vi "Main.vi"() -> ()   [LabVIEW 2013]
doc: "This template is for the Queued Message Handler design pattern.\n\nThe Event Handling Loop generates messages based on user interface actions.\n\nThe Message Handling Loop processes messages generated by the Event Handling Loop, or by other messages. The messages are string values, so new messages can be added easily to the Message Cases case structure in the Message Handling Loop. Each message cluster can also provide an optional value for Message Data, which is a variant that can be converted to whatever message-specific data is required."
uses:
  controls/UI Data.ctl
  <vilib>/addons/zeromq/socket_type.ctl
  <vilib>/addons/zeromq/socket_options.ctl
  controls/JSON RPC Request.ctl
  controls/JSON RPC Response.ctl
  support/Message Queue/Enqueue Message (Array).vi
  support/Message Queue/Enqueue Message (Single).vi
  <vilib>/Utility/error.llb/Error Cluster From Error Code.vi
  <vilib>/ErrorRing/Error Ring.xnode
  support/Message Queue/Message Queue.lvlib
  support/User Event - Stop/User Event - Stop.lvlib
  <vilib>/addons/zeromq/zmq_context.lvclass
  <vilib>/addons/zeromq/zeromq.lvlib
  <vilib>/addons/zeromq/zmq_socket.lvclass
panel:
  out "Display <Replace Me>":string
  in  "Do Something Else <Replace Me>":bool
  in  "Do Something <Replace Me>":bool
  in  "Exit":bool
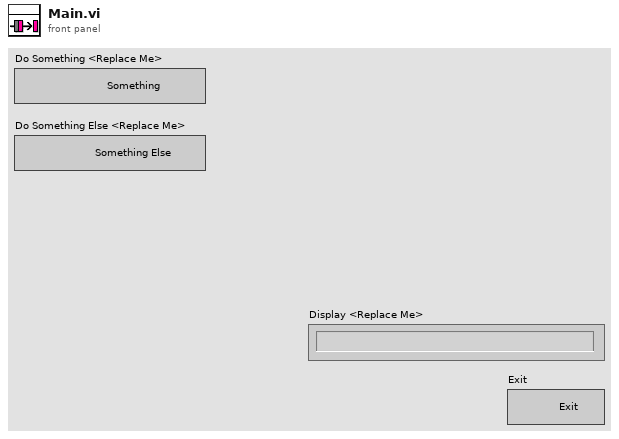
[diagram p1: front panel]
types:
  T1 = typedef "zeromq.lvlib/socket_options.ctl" = enum8{"NONE", "ZMQ_HWM", "<2>", "ZMQ_SWAP", "ZMQ_AFFINITY", "ZMQ_IDENTITY", "ZMQ_SUBSCRIBE", "ZMQ_UNSUBSCRIBE", "ZMQ_RATE", "ZMQ_RECOVERY_IVL", "ZMQ_MCAST_LOOP", "ZMQ_SNDBUF", "ZMQ_RCVBUF", "ZMQ_RCVMORE", "ZMQ_FD", "ZMQ_EVENTS", "ZMQ_TYPE", "ZMQ_LINGER", "ZMQ_RECONNECT_IVL", "ZMQ_BACKLOG", "ZMQ_RECOVERY_IVL_MSEC", "ZMQ_RECONNECT_IVL_MAX", "ZMQ_MAXMSGSIZE", "ZMQ_SNDHWM", "ZMQ_RCVHWM", "ZMQ_MULTICAST_HOPS", "<26>", "ZMQ_RCVTIMEO", "ZMQ_SNDTIMEO", "<29>", "<30>", "ZMQ_IPV4ONLY", "ZMQ_LAST_ENDPOINT", "ZMQ_ROUTER_MANDATORY", "ZMQ_TCP_KEEPALIVE", "ZMQ_TCP_KEEPALIVE_CNT", "ZMQ_TCP_KEEPALIVE_IDLE", "ZMQ_TCP_KEEPALIVE_INTVL", "ZMQ_TCP_ACCEPT_FILTER", "ZMQ_DELAY_ATTACH_ON_CONNECT", "ZMQ_XPUB_VERBOSE"}
  T2 = typedef "zeromq.lvlib/socket_type.ctl" = enum8{"ZMQ_PAIR", "ZMQ_PUB", "ZMQ_SUB", "ZMQ_REQ", "ZMQ_REP", "ZMQ_DEALER", "ZMQ_ROUTER", "ZMQ_PULL", "ZMQ_PUSH", "ZMQ_XPUB", "ZMQ_XSUB"}
  T3 = typedef "UI Data.ctl" = cluster{"Boolean <Replace Me>":bool, "String <Replace Me>":string, "Numeric <Replace Me>":dbl, "Do Something Ref":refnum<vi>, "Do Something Else Ref":refnum<vi>, "Data Display Ref":refnum<vi>, "Exit Button Ref":refnum<vi>}
  T4 = typedef "Message Queue.lvlib/All Message Queues.ctl" = cluster{"UI":refnum<queue>}
  T5 = typedef "JSON RPC Request.ctl" = cluster{"id":dbl, "method":string, "jsonrpc":string, "params":string}
  T6 = typedef "JSON RPC Response.ctl" = cluster{"id":dbl, "result":string, "jsonrpc":string}
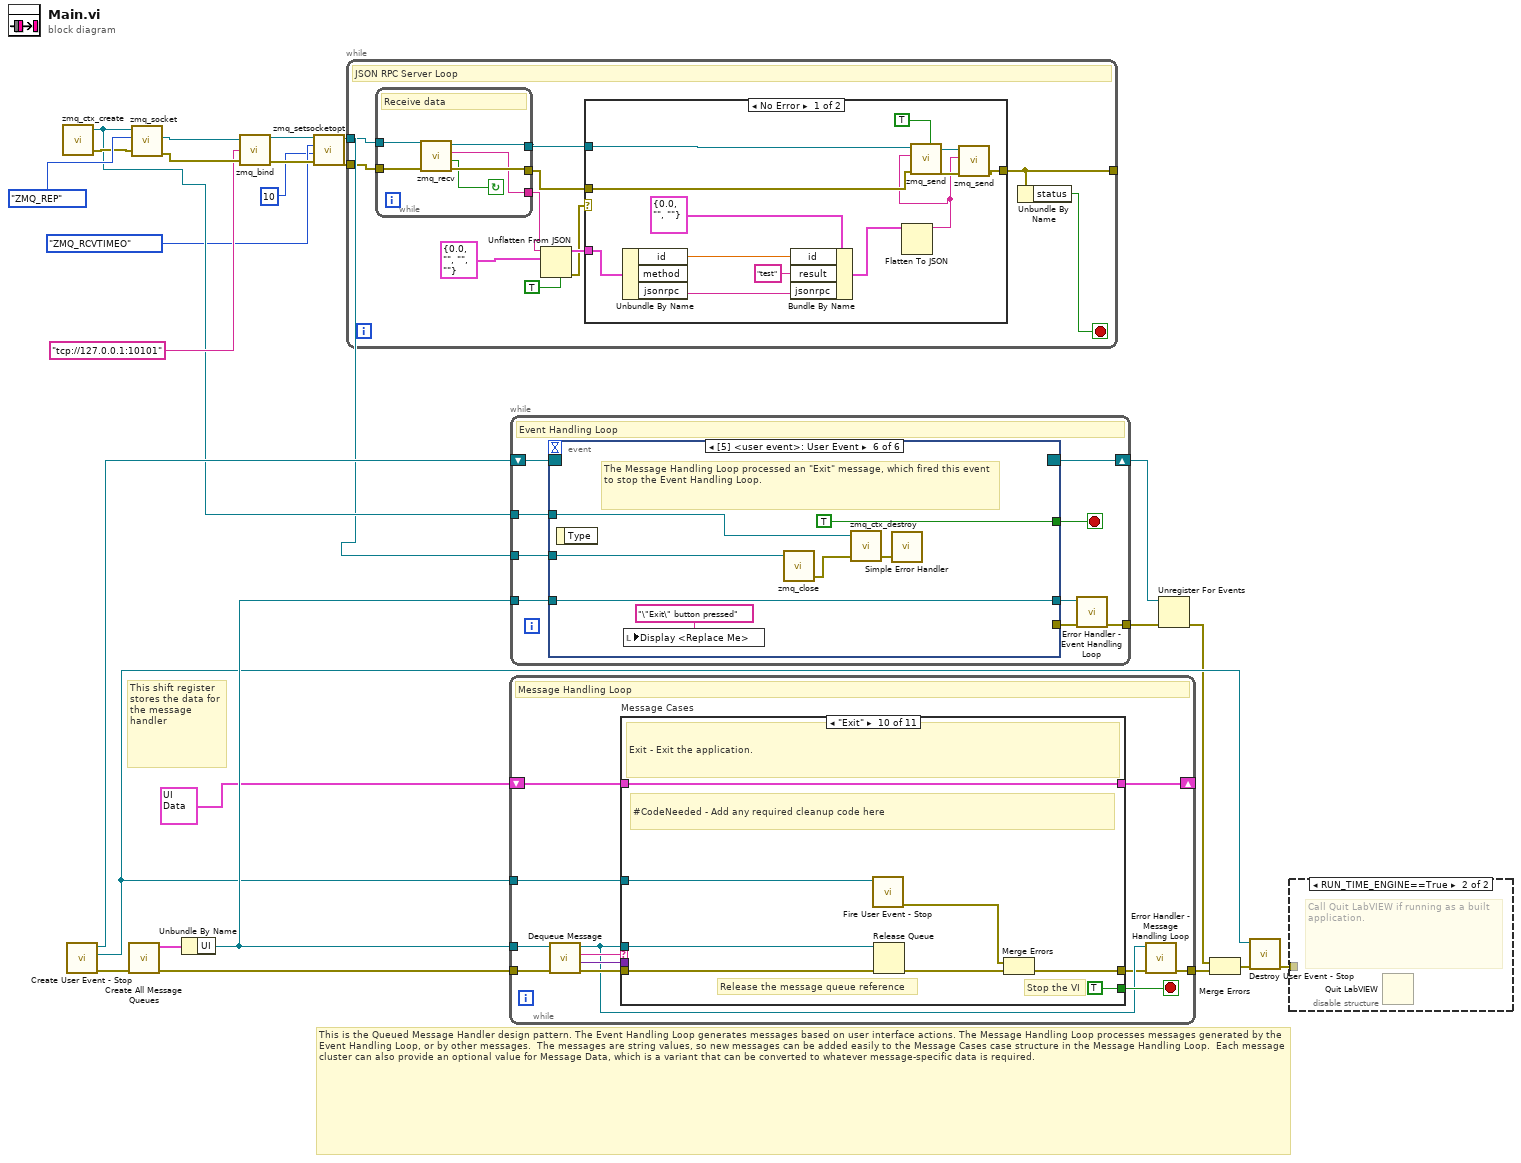
[diagram p0: block diagram]
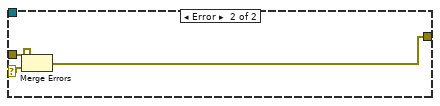
[diagram p2: hidden frame]
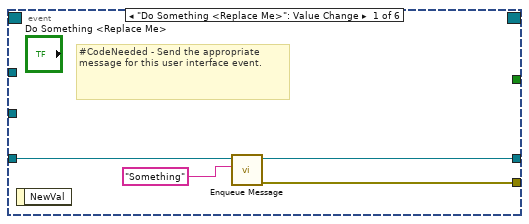
[diagram p4: hidden frame]
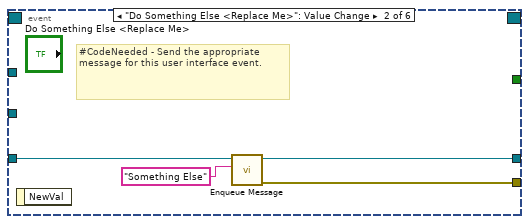
[diagram p5: hidden frame]
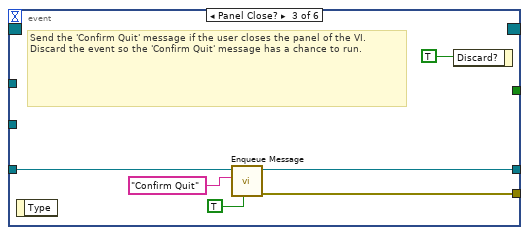
[diagram p6: hidden frame]
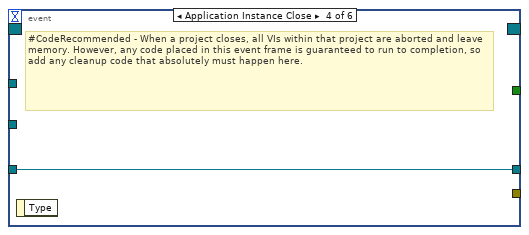
[diagram p7: hidden frame]
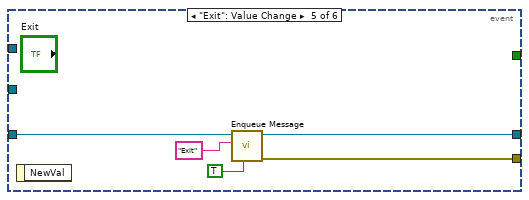
[diagram p8: hidden frame]
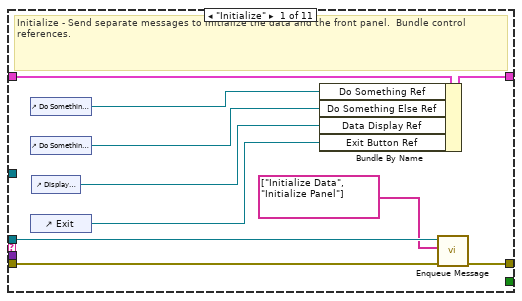
[diagram p9: hidden frame]
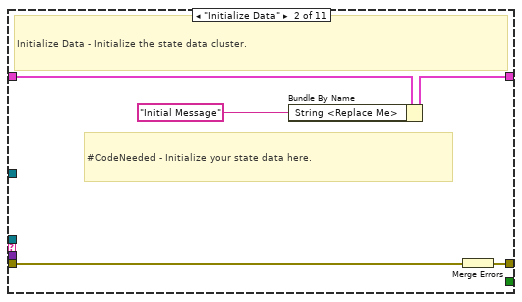
[diagram p10: hidden frame]
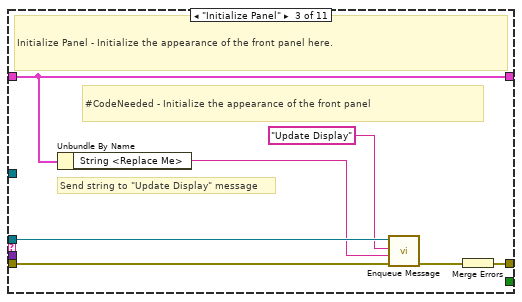
[diagram p11: hidden frame]
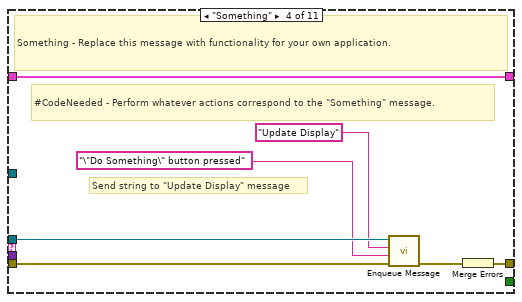
[diagram p12: hidden frame]
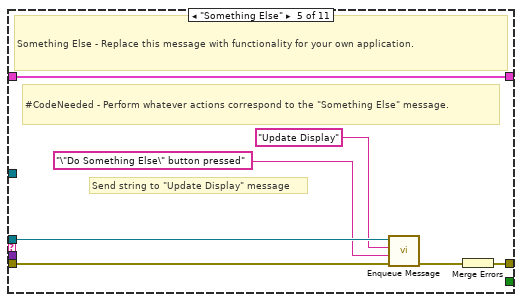
[diagram p13: hidden frame]
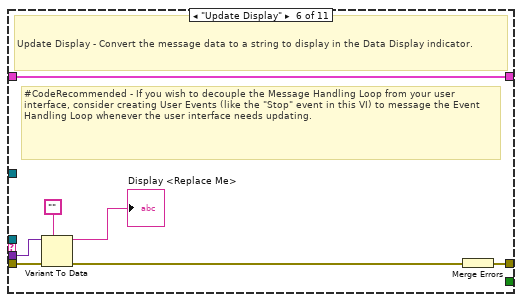
[diagram p14: hidden frame]
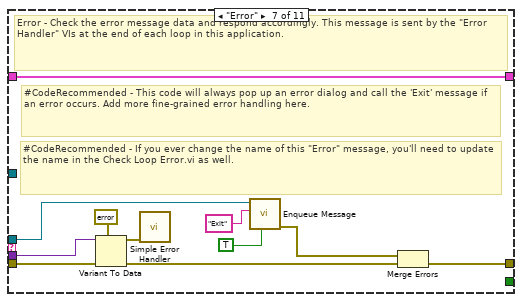
[diagram p15: hidden frame]
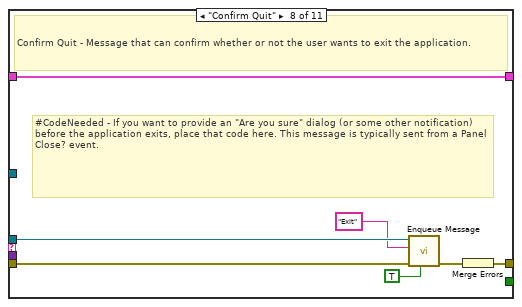
[diagram p16: hidden frame]
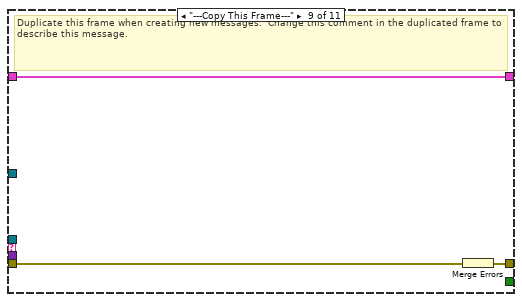
[diagram p17: hidden frame]
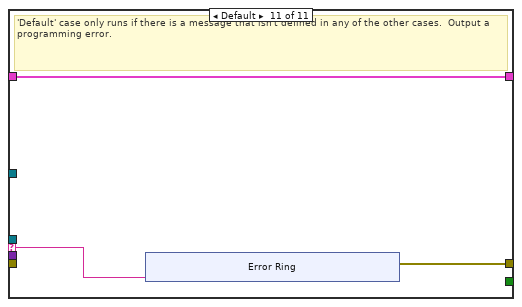
[diagram p18: hidden frame]
diagram:
  # "This is the Queued Message Handler design pattern. The Event Handling Loop generates messages based on user interface actions. The Message Handling Loop processes messages generated by the Event Handling Loop, or by other messages.  The messages are string values, so new messages can be added easily to the Message Cases case structure in the Message Handling Loop.  Each message cluster can also provide an optional value for Message Data, which is a variant that can be converted to whatever message-specific data is required."
  # "This shift register stores the data for the message handler"
  n1 = call <vilib>:"zmq_ctx_create.vi"() -> ("error out"=w11:errorcluster, "context out"=w7:refnum<class "zmq_context.lvclass">)  [unwired: 4 in]
  n2 = call "Create User Event - Stop.vi"() -> ("error out"=w20:errorcluster, "User Event - Stop"=w18:refnum<user-event>, "Stop Event Registration Refnum"=w21:refnum<event-registration>)  [unwired: 9 in]
  n3 = call "Create All Message Queues.vi"("error in (no error)"=w20) -> ("error out"=w25:errorcluster, "Message Queues out"=w24:T4)  [unwired: 9 in]
  n4 = call <vilib>:"zmq_socket.vi"("error in"=w11, "socket type"=socket_type."ZMQ_REP", "context in"=w7) -> ("error out"=w10:errorcluster, "socket out"=w9:refnum<class "zmq_socket.lvclass">)  [unwired: 2 in, 1 out]
  n5 = Unbundle By Name(w24) -> ("UI"=w22:refnum<queue>)
  n6 = call <vilib>:"zmq_bind.vi"("error in"=w10, "endpoint"="tcp://127.0.0.1:10101", "socket in"=w9) -> ("error out"=w5:errorcluster, "socket out"=w6:refnum<class "zmq_socket.lvclass">)  [unwired: 1 in]
  n7 = call <vilib>:"zmq_setsocketopt.vi"("error in"=w5, "value"=10, "option"=socket_options."ZMQ_RCVTIMEO", "socket in"=w6) -> ("error out"=w2:errorcluster, "socket out"=w1:refnum<class "zmq_socket.lvclass">)  [unwired: 2 in]
  n8 = while {
    tunnel: [w32] -> _
    tunnel: w1 -> [w35]
    tunnel: w2 -> [w34]
    stop <- w31 stop-if-true
    # "JSON RPC Server Loop"
    n9 = while {
      tunnel: [w58] -> w33
      tunnel: [w57] -> w36
      tunnel: w35 -> [w55]
      tunnel: w34 -> [w54]
      tunnel: [w53] -> w30
      stop <- w56 continue-if-true
      # "Receive data"
      n10 = call <vilib>:"zmq_recv.vi"("error in"=w54, "socket in"=w55) -> ("error out"=w58:errorcluster, "more?"=w56:bool, "data"=w53:string, "socket out"=w57:refnum<class "zmq_socket.lvclass">)  [unwired: 3 in, 1 out]
    }
    n11 = Unflatten From JSON(JSON string=w30, type and defaults=T5 {"id"=0.0, "method"="", "jsonrpc"="", "params"=""} ("JSON RPC Request"), strict validation? (F)=TRUE) -> (value=w28:T5, error out=w26:errorcluster)  [unwired: 4 in]
    n12 = case shown="No Error" w26 {
      selector: w26 -> [_ w52]
      tunnel: w36 -> [w49 _]
      tunnel: w33 -> [w48 w51]
      tunnel: [w47 w50] -> w32
      tunnel: w28 -> [w46 _]
      frame No Error {
        n13 = Unbundle By Name(w46) -> ("id"=w39:dbl, "jsonrpc"=w40:string)  [unwired: 1 out]
        n14 = Bundle By Name(cluster=T6 {"id"=0.0, "result"="", "jsonrpc"=""} ("JSON RPC Response"), "id"=w39, "result"="test", "jsonrpc"=w40) -> (w41:T6)
        n15 = Flatten To JSON(anything=w41) -> (JSON string=w37:string)  [unwired: 2 in, 1 out]
        n16 = call <vilib>:"zmq_send.vi"("error in"=w48, "data"=w37, "socket in"=w49, "more? (F)"=TRUE) -> ("error out"=w43:errorcluster, "socket out"=w44:refnum<class "zmq_socket.lvclass">)  [unwired: 3 in]
        n17 = call <vilib>:"zmq_send.vi"("error in"=w43, "data"=w37, "socket in"=w44) -> ("error out"=w47:errorcluster)  [unwired: 4 in, 1 out]
      }
      frame Error {
        n18 = Merge Errors(w51, w52) -> (w50:errorcluster)
      }
    }
    n19 = Unbundle By Name(w32) -> ("status"=w31:bool)
  }
  n20 = while {
    tunnel: w22 -> [w62]
    shift-right: [w69] -> _
    shift-left: T3 {"Boolean <Replace Me>"=FALSE, "String <Replace Me>"="", "Numeric <Replace Me>"=0.0, "Do Something Ref"=refnum, "Do Something Else Ref"=refnum, "Data Display Ref"=refnum, "Exit Button Ref"=refnum} ("Data Cluster") -> [w70]
    tunnel: w18 -> [w67]
    tunnel: w25 -> [w66]
    tunnel: [w60] -> w23
    stop <- w68 stop-if-true
    # "Message Handling Loop"
    n21 = call "Dequeue Message.vi"("error in (no error)"=w66, "Message Queue"=w62) -> ("error out"=w65:errorcluster, "Message Data"=w63:variant, "Message"=w64:string, "dup Message Queue"=w61:refnum<queue>)  [unwired: 6 in]
    n22 = case "Message Cases" shown="\"Exit\"" w64 {
      selector: w64 -> [_ _ _ _ _ _ _ _ _ _ w143]
      tunnel: w61 -> [w78 _ w89 w95 w102 _ w116 w127 _ w142 _]
      tunnel: w65 -> [w79 w85 w90 w97 w104 w111 w124 w131 w134 w137 _]
      tunnel: [w80 w81 w91 w98 w105 w112 w117 w129 w132 w138 w144] -> w59
      tunnel: w70 -> [w77 w84 w92 w99 w106 w113 w123 w130 w133 w141 w145]
      tunnel: [w76 w83 w92 w99 w106 w113 w123 w130 w133 w141 w145] -> w69
      tunnel: [_ _ _ _ _ _ _ _ _ TRUE _] -> w68
      tunnel: w63 -> [_ _ _ _ _ w110 w122 _ _ _ _]
      tunnel: w67 -> [_ _ _ _ _ _ _ _ _ w136 _]
      frame "Initialize" {
        # "Initialize - Send separate messages to initialize the data and the front panel.  Bundle control references."
        n23 = control-ref of="Do Something <Replace Me>"() -> (w75:refnum<vi>)
        n24 = control-ref of="Do Something Else <Replace Me>"() -> (w74:refnum<vi>)
        n25 = control-ref of="Exit"() -> (w72:refnum<vi>)
        n26 = control-ref of="Display <Replace Me>"() -> (w73:refnum<vi>)
        n27 = Bundle By Name(cluster=w77, "Do Something Ref"=w75, "Do Something Else Ref"=w74, "Data Display Ref"=w73, "Exit Button Ref"=w72) -> (w76:T3)
        n28 = call-poly "Enqueue Message.vi"("error in (no error)"=w79, "Message Array"=string[] ["Initialize Data", "Initialize Panel"], "Message Queue"=w78) -> ("error out"=w80:errorcluster)  [unwired: 7 in, 1 out]
      }
      frame "Initialize Data" {
        # "#CodeNeeded - Initialize your state data here."
        # "Initialize Data - Initialize the state data cluster."
        n29 = Bundle By Name(cluster=w84, "String <Replace Me>"="Initial Message" ("Initial Message")) -> (w83:T3)
        n30 = Merge Errors(w85) -> (w81:errorcluster)
      }
      frame "Initialize Panel" {
        # "Send string to \"Update Display\" message"
        # "#CodeNeeded - Initialize the appearance of the front panel"
        # "Initialize Panel - Initialize the appearance of the front panel here."
        n31 = Unbundle By Name(w92) -> ("String <Replace Me>"=w86:string)
        n32 = call-poly "Enqueue Message.vi"("error in (no error)"=w90, "Message Data"=w86, "Message"="Update Display", "Message Queue"=w89) -> ("error out"=w88:errorcluster)  [unwired: 6 in, 1 out]
        n33 = Merge Errors(w88) -> (w91:errorcluster)
      }
      frame "Something" {
        # "Send string to \"Update Display\" message"
        # "#CodeNeeded - Perform whatever actions correspond to the \"Something\" message."
        # "Something - Replace this message with functionality for your own application."
        n34 = call-poly "Enqueue Message.vi"("error in (no error)"=w97, "Message Data"="\"Do Something\" button pressed" ("\"Do Something\" button pressed"), "Message"="Update Display", "Message Queue"=w95) -> ("error out"=w96:errorcluster)  [unwired: 6 in, 1 out]
        n35 = Merge Errors(w96) -> (w98:errorcluster)
      }
      frame "Something Else" {
        # "Send string to \"Update Display\" message"
        # "#CodeNeeded - Perform whatever actions correspond to the \"Something Else\" message."
        # "Something Else - Replace this message with functionality for your own application."
        n36 = call-poly "Enqueue Message.vi"("error in (no error)"=w104, "Message Data"="\"Do Something Else\" button pressed" ("\"Do Something Else\" button pressed"), "Message"="Update Display", "Message Queue"=w102) -> ("error out"=w103:errorcluster)  [unwired: 6 in, 1 out]
        n37 = Merge Errors(w103) -> (w105:errorcluster)
      }
      frame "Update Display" {
        # "#CodeRecommended - If you wish to decouple the Message Handling Loop from your user interface, consider creating User Events (like the \"Stop\" event in this VI) to message the Event Handling Loop whenever the user interface needs updating."
        # "Update Display - Convert the message data to a string to display in the Data Display indicator."
        n38 = Variant To Data(error in=w111, type="", Variant=w110) -> (data=→"Display <Replace Me>":string, error out=w108:errorcluster)
        n39 = Merge Errors(w108) -> (w112:errorcluster)
      }
      frame "Error" {
        # "#CodeRecommended - If you ever change the name of this \"Error\" message, you'll need to update the name in the Check Loop Error.vi as well."
        # "#CodeRecommended - This code will always pop up an error dialog and call the 'Exit' message if an error occurs. Add more fine-grained error handling here."
        # "Error - Check the error message data and respond accordingly. This message is sent by the \"Error Handler\" VIs at the end of each loop in this application."
        n40 = Variant To Data(error in=w124, type=errorcluster {"status"=FALSE, "code"=0, "source"=""} ("error constant"), Variant=w122) -> (data=w120:errorcluster, error out=w119:errorcluster)
        n41 = call <vilib>:"Simple Error Handler.vi"("error in (no error)"=w120) -> ()  [unwired: 4 in, 5 out]
        n42 = call-poly "Enqueue Message.vi"("Priority Message? (F)"=TRUE, "Message"="Exit", "Message Queue"=w116) -> ("error out"=w118:errorcluster)  [unwired: 7 in, 1 out]
        n43 = Merge Errors(w118, w119) -> (w117:errorcluster)
      }
      frame "Confirm Quit" {
        # "#CodeNeeded - If you want to provide an \"Are you sure\" dialog (or some other notification) before the application exits, place that code here. This message is typically sent from a Panel Close? event."
        # "Confirm Quit - Message that can confirm whether or not the user wants to exit the application."
        n44 = call-poly "Enqueue Message.vi"("Priority Message? (F)"=TRUE, "error in (no error)"=w131, "Message"="Exit", "Message Queue"=w127) -> ("error out"=w128:errorcluster)  [unwired: 6 in, 1 out]
        n45 = Merge Errors(w128) -> (w129:errorcluster)
      }
      frame "---Copy This Frame---" {
        # "Duplicate this frame when creating new messages.  Change this comment in the duplicated frame to describe this message."
        n46 = Merge Errors(w134) -> (w132:errorcluster)
      }
      frame "Exit" {
        # "Stop the VI"
        # "Release the message queue reference"
        # "#CodeNeeded - Add any required cleanup code here"
        # "Exit - Exit the application."
        n47 = call "Fire User Event - Stop.vi"("User Event - Stop"=w136) -> ("error out"=w135:errorcluster)  [unwired: 10 in]
        n48 = Release Queue(queue=w142, error in (no error)=w137) -> (error out=w139:errorcluster)  [unwired: 1 in, 2 out]
        n49 = Merge Errors(w135, w139) -> (w138:errorcluster)
      }
      frame Default {
        # "'Default' case only runs if there is a message that isn't defined in any of the other cases.  Output a programming error."
        n50 = xnode "Error Ring"("parameter 0"=w143) -> ("error out"=w144:errorcluster)
      }
    }
    n51 = call "Error Handler - Message Handling Loop.vi"("error in (no error)"=w59, "Message Queue"=w61) -> ("dup error in"=w60:errorcluster)  [unwired: 8 in, 1 out]
  }
  n52 = while {
    tunnel: w22 -> [w161]
    shift-right: [w159] -> w16
    shift-left: w21 -> [w160]
    tunnel: [w155] -> w13
    tunnel: w7 -> [w154]
    tunnel: w1 -> [w153]
    stop <- w157 stop-if-true
    # "Event Handling Loop"
    n53 = event shown="[5] <user event>: User Event" {
      selector: w160 -> [_ _ _ _ _ _]
      dyn-events: [_ _ _ _ _ _] -> w159
      timeout: _ -> [_ _ _ _ _ _]
      tunnel: [_ _ _ _ _ TRUE ("Discard?")] -> w157
      tunnel: w161 -> [w165 w169 w174 w176 w181 w188]
      tunnel: [w162 w166 w173 _ w180 _] -> w158
      tunnel: [w164 w168 w172 w176 w179 w188] -> w156
      tunnel: w154 -> [_ _ _ _ _ w183]
      tunnel: w153 -> [_ _ _ _ _ w182]
      event "Do Something <Replace Me>": Value Change {
        # "#CodeNeeded - Send the appropriate message for this user interface event."
        n54 = event-data() -> ()  [unwired: 1 in, 1 out]
        n55 = call-poly "Enqueue Message.vi"("Message"="Something", "Message Queue"=w165) -> ("error out"=w162:errorcluster, "dup Message Queue"=w164:refnum<queue>)  [unwired: 8 in]
      }
      event "Do Something Else <Replace Me>": Value Change {
        # "#CodeNeeded - Send the appropriate message for this user interface event."
        n56 = event-data() -> ()  [unwired: 1 in, 1 out]
        n57 = call-poly "Enqueue Message.vi"("Message"="Something Else", "Message Queue"=w169) -> ("error out"=w166:errorcluster, "dup Message Queue"=w168:refnum<queue>)  [unwired: 8 in]
      }
      event Panel Close? {
        # "Send the 'Confirm Quit' message if the user closes the panel of the VI. Discard the event so the 'Confirm Quit' message has a chance to run."
        n58 = event-data() -> ()  [unwired: 1 in, 1 out]
        n59 = call-poly "Enqueue Message.vi"("Priority Message? (F)"=TRUE, "Message"="Confirm Quit", "Message Queue"=w174) -> ("error out"=w173:errorcluster, "dup Message Queue"=w172:refnum<queue>)  [unwired: 7 in]
        n60 = event-data("Discard?"=TRUE) -> ()  [unwired: 1 in, 1 out]
      }
      event Application Instance Close {
        # "#CodeRecommended - When a project closes, all VIs within that project are aborted and leave memory. However, any code placed in this event frame is guaranteed to run to completion, so add any cleanup code that absolutely must happen here."
        n61 = event-data() -> ()  [unwired: 1 in, 1 out]
      }
      event "Exit": Value Change {
        n62 = event-data() -> ()  [unwired: 1 in, 1 out]
        n63 = call-poly "Enqueue Message.vi"("Priority Message? (F)"=TRUE, "Message"="Exit", "Message Queue"=w181) -> ("error out"=w180:errorcluster, "dup Message Queue"=w179:refnum<queue>)  [unwired: 7 in]
      }
      event User Event {
        # "The Message Handling Loop processed an \"Exit\" message, which fired this event to stop the Event Handling Loop."
        n64 = event-data() -> ()  [unwired: 1 in, 1 out]
        n65 = local write "Display <Replace Me>"("\"Exit\" button pressed" ("VI Stopped")) -> ()
        n66 = call <vilib>:"zmq_close.vi"("socket"=w182) -> ("error out"=w185:errorcluster)  [unwired: 4 in]
        n67 = call <vilib>:"zmq_ctx_destroy.vi"("error in"=w185, "context in"=w183) -> ("error out"=w184:errorcluster)  [unwired: 3 in]
        n68 = call <vilib>:"Simple Error Handler.vi"("error in (no error)"=w184) -> ()  [unwired: 4 in, 5 out]
      }
    }
    n69 = call "Error Handler - Event Handling Loop.vi"("error in (no error)"=w158, "Message Queue"=w156) -> ("dup error in"=w155:errorcluster)  [unwired: 8 in, 1 out]
  }
  n70 = Unregister For Events(event registration refnum=w16, error in=w13) -> (error out=w17:errorcluster)
  n71 = Merge Errors(w17, w23) -> (w19:errorcluster)
  n72 = call "Destroy User Event - Stop.vi"("error in (no error)"=w19, "User Event - Stop"=w18) -> ("error out"=w14:errorcluster)  [unwired: 9 in]
  n73 = disable-structure shown="RUN_TIME_ENGINE==True" {
    disable-tunnel: w14 -> [_ _]
    frame condition #0 (active) {
    }
    frame condition #1 {
      # "Call Quit LabVIEW if running as a built application."
      n74 = Quit LabVIEW() -> ()  [unwired: 1 in]
    }
  }
